vi "GUI Init.vi"(8 "error in (no error)":errorcluster, 10 "GUI Refs":T1, 11 "View Model":T2) -> (0 "error out":errorcluster, 3 "View Model":T2)   [LabVIEW 2017]
doc: "Initialize all GUI Arrays of all used modules"
uses:
  View Model/Controls/View Model.ctl
  View Model/Controls/Shared Model.ctl
  Error Handler/Controls/Error Model.ctl
  Error Handler/Controls/Error Event.ctl
  Error Handler/Controls/Error Type.ctl
  Controller/Controls/Controller Model.ctl
  Controller/Controls/Controller Event.ctl
  Controller/Controls/Controller Command.ctl
  Controller/Controls/Controller Overhead.ctl
  Real-Time/RT Status.ctl
  Real-Time/RT Loop Status.ctl
  Controller/Controls/Controller NStream.ctl
  Controller/Controls/Controller Timer Data.ctl
  Controller/Controls/Controller DAQ Data.ctl
  TDMS Logger/Controls/TDMS Model.ctl
  TDMS Logger/Controls/TDMS Event.ctl
  TDMS Logger/Controls/TDMS Command.ctl
  TDMS Logger/Controls/TDMS Overhead.ctl
  TDMS Logger/Controls/TDMS ChanProperties.ctl
  TDMS Logger/Controls/TDMS DAQ Data.ctl
  Controls/GUI Referencies.ctl
  Controls/TDMS_GUI_Cluster.ctl
  Controls/AIMV_GUI_Cluster.ctl
  Controls/AOM_GUI_Cluster.ctl
  Controls/Discrete_GUI_Cluster.ctl
  GUI Init - DOM6.vi
  GUI Init - DIM4.vi
  GUI Init - DIM3.vi
  GUI Init - AIMC.vi
  GUI Init - AIMV.vi
  GUI Init - AOM.vi
  GUI Init - DOM7.vi
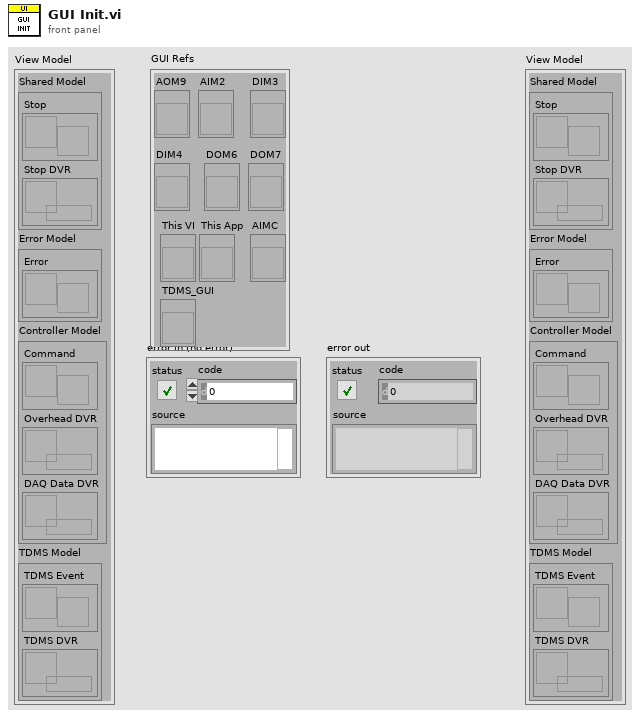
[diagram p1: front panel]
types:
  T1 = typedef "GUI Referencies.ctl" = cluster{"This VI":refnum<vi>, "This App":refnum<vi>, "DIM3":refnum<vi>, "DIM4":refnum<vi>, "DOM6":refnum<vi>, "DOM7":refnum<vi>, "AOM9":refnum<vi>, "AIM2":refnum<vi>, "AIMC":refnum<vi>, "TDMS_GUI":refnum<vi>}
  T2 = typedef "View Model.ctl" = cluster{"Shared Model":T3, "Error Model":T4, "Controller Model":T5, "TDMS Model":T6}
  T3 = typedef "Shared Model.ctl" = cluster{"Stop":refnum<user-event>, "Stop DVR":refnum<data-value>}
  T4 = typedef "Error Model.ctl" = cluster{"Error":refnum<user-event>}
  T5 = typedef "Controller Model.ctl" = cluster{"Command":refnum<user-event>, "Overhead DVR":refnum<data-value>, "DAQ Data DVR":refnum<data-value>}
  T6 = typedef "TDMS Model.ctl" = cluster{"TDMS Event":refnum<user-event>, "TDMS DVR":refnum<data-value>}
  T7 = enum8{"Enabled", "Disabled", "Disabled and Grayed Out"}
  T8 = typedef "Controller DAQ Data.ctl" = cluster{"AOM data":dbl[], "AIMV data":dbl[], "AIMC data":dbl[], "DOM data":dbl[], "DIM data":dbl[], "AOM timestamp":dbl, "AIMV timestamp":dbl, "AIMC timestamp":dbl, "DOM timestamp":dbl, "DIM timestamp":dbl}
  T9 = typedef "AIMV_GUI_Cluster.ctl" = cluster{"Ch.name":string, "Ch.value":dbl, "Ch.range":string, "Num":string}
  T10 = typedef "Discrete_GUI_Cluster.ctl" = cluster{"Ch.name":string, "Ch.state":bool, "Num":string}
  T11 = typedef "AOM_GUI_Cluster.ctl" = cluster{"Ch.name":string, "Ch.value":dbl, "Ch.mode":enum16{"0-5 V", "+/-10 V", "0-5 mA", "4-20 mA"}, "Num":string}
  T12 = typedef "TDMS ChanProperties.ctl" = cluster{"AOM9":string[][], "AIM2":string[][], "DIM3":string[][], "DIM4":string[][], "DOM6":string[][], "DOM7":string[][]}
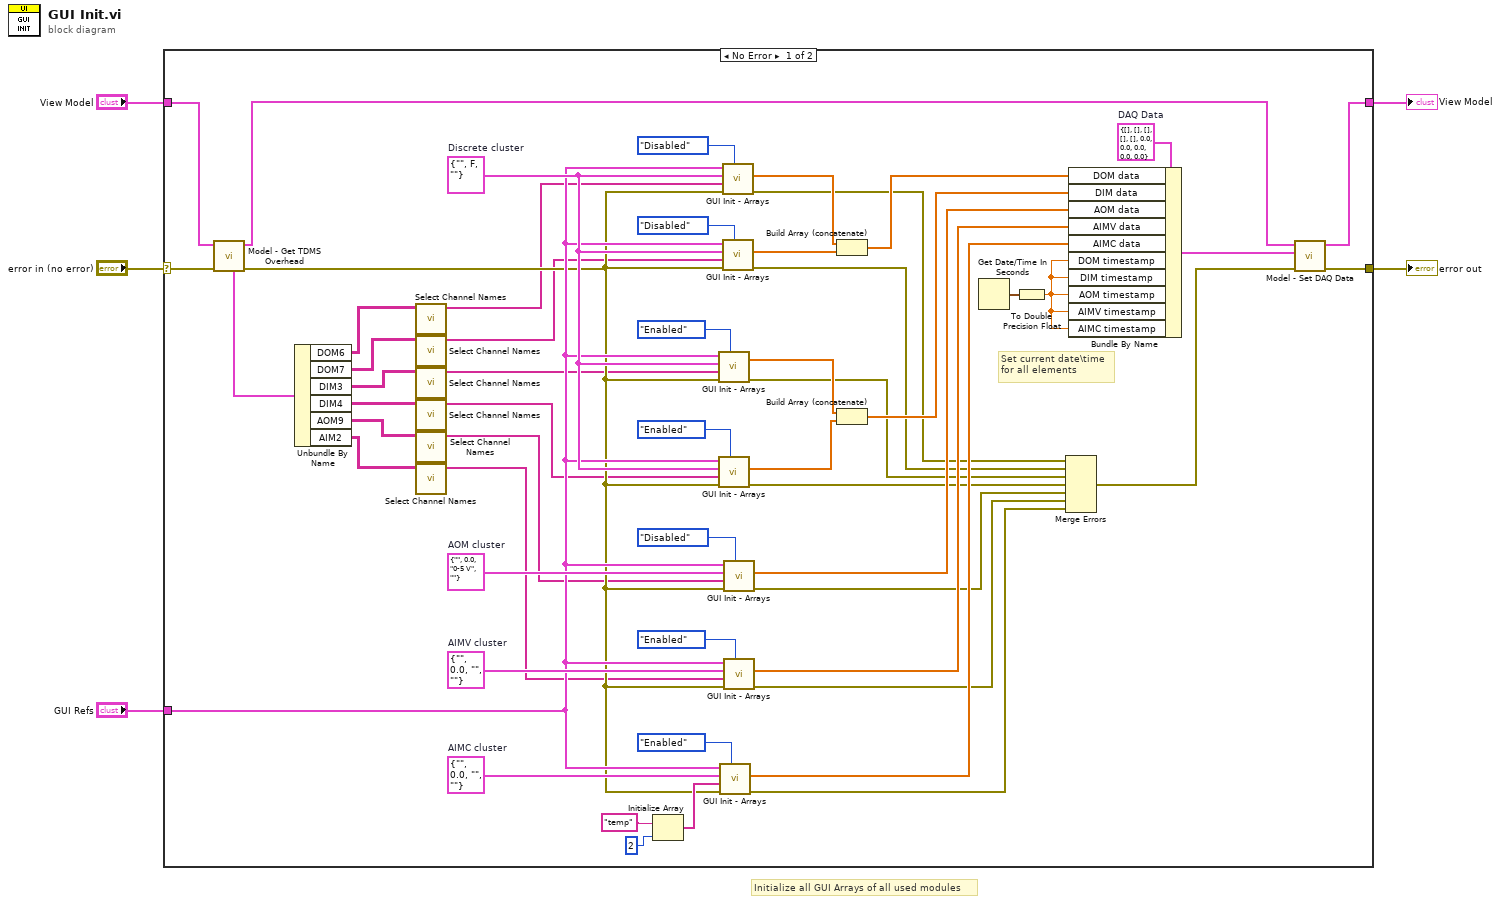
[diagram p0: block diagram]
diagram:
  # "Initialize all GUI Arrays of all used modules"
  n1 = case shown="No Error" "error in (no error)" {
    selector: "error in (no error)" -> [w33 w61]
    tunnel: [w51 w61] -> w4
    tunnel: "View Model" -> [w36 w62]
    tunnel: [w53 w62] -> w2
    tunnel: "GUI Refs" -> [w37 _]
    frame No Error {
      w57 = T8 {"AOM data"=[], "AIMV data"=[], "AIMC data"=[], "DOM data"=[], "DIM data"=[], "AOM timestamp"=0.0, "AIMV timestamp"=0.0, "AIMC timestamp"=0.0, "DOM timestamp"=0.0, "DIM timestamp"=0.0}  # DAQ Data
      w59 = T9 {"Ch.name"="", "Ch.value"=0.0, "Ch.range"="", "Num"=""}  # AIMV cluster
      w47 = T10 {"Ch.name"="", "Ch.state"=FALSE, "Num"=""}  # Discrete cluster
      w60 = T11 {"Ch.name"="", "Ch.value"=0.0, "Ch.mode"=enum."0-5 V", "Num"=""}  # AOM cluster
      w58 = T9 {"Ch.name"="", "Ch.value"=0.0, "Ch.range"="", "Num"=""}  # AIMC cluster
      # "Set current date\\time\nfor all elements"
      n2 = call "Model - Get TDMS Overhead.vi"("error in (no error)"=w33, "View Model"=w36) -> ("error out"=w32:errorcluster, "View Model"=w35:T2, "ChProps"=w34:T12)  [unwired: 4 in, 3 out]
      n3 = Unbundle By Name(w34) -> ("DOM6"=w17:string[][], "DOM7"=w16:string[][], "DIM3"=w15:string[][], "DIM4"=w14:string[][], "AOM9"=w13:string[][], "AIM2"=w12:string[][])
      n4 = call "Select Channel Names.vi"("2D Channel Params"=w17) -> ("Ch.Description -1"=w11:string[])  [unwired: 8 in, 2 out]
      n5 = call "Select Channel Names.vi"("2D Channel Params"=w16) -> ("Ch.Description -1"=w10:string[])  [unwired: 8 in, 2 out]
      n6 = call "Select Channel Names.vi"("2D Channel Params"=w15) -> ("Ch.Description -1"=w9:string[])  [unwired: 8 in, 2 out]
      n7 = call "Select Channel Names.vi"("2D Channel Params"=w14) -> ("Ch.Description -1"=w8:string[])  [unwired: 8 in, 2 out]
      n8 = call "Select Channel Names.vi"("2D Channel Params"=w13) -> ("Ch.Description -1"=w7:string[])  [unwired: 8 in, 2 out]
      n9 = call "Select Channel Names.vi"("2D Channel Params"=w12) -> ("Ch.Description -1"=w6:string[])  [unwired: 8 in, 2 out]
      n10 = Initialize Array("temp" ("Ch.range"), 2 ("dimension size")) -> (w44:string[])
      n11 = call-poly "GUI Init - Arrays.vi"("Disabled"=T7."Enabled", "error in (no error)"=w32, "Ch.names"=w9, "Cluster"=w47, "GUI Refs"=w37) -> ("error out"=w20:errorcluster, "Data"=w39:dbl[])  [unwired: 4 in, 1 out]
      n12 = call-poly "GUI Init - Arrays.vi"("Disabled"=T7."Enabled", "error in (no error)"=w32, "Ch.names"=w8, "Cluster"=w47, "GUI Refs"=w37) -> ("error out"=w21:errorcluster, "Data"=w40:dbl[])  [unwired: 4 in, 1 out]
      n13 = call-poly "GUI Init - Arrays.vi"("Disabled"=T7."Enabled", "error in (no error)"=w32, "Ch.names"=w44, "Cluster"=w58, "GUI Refs"=w37) -> ("error out"=w31:errorcluster, "Data"=w50:dbl[])  [unwired: 4 in, 1 out]
      n14 = call-poly "GUI Init - Arrays.vi"("Disabled"=T7."Disabled", "error in (no error)"=w32, "Ch.names"=w11, "Cluster"=w47, "GUI Refs"=w37) -> ("error out"=w18:errorcluster, "Data"=w43:dbl[])  [unwired: 4 in, 1 out]
      n15 = call-poly "GUI Init - Arrays.vi"("Disabled"=T7."Disabled", "error in (no error)"=w32, "Ch.names"=w10, "Cluster"=w47, "GUI Refs"=w37) -> ("error out"=w19:errorcluster, "Data"=w42:dbl[])  [unwired: 4 in, 1 out]
      n16 = call-poly "GUI Init - Arrays.vi"("Disabled"=T7."Disabled", "error in (no error)"=w32, "Ch.names"=w7, "Cluster"=w60, "GUI Refs"=w37) -> ("error out"=w29:errorcluster, "Data"=w48:dbl[])  [unwired: 4 in, 1 out]
      n17 = call-poly "GUI Init - Arrays.vi"("Disabled"=T7."Enabled", "error in (no error)"=w32, "Ch.names"=w6, "Cluster"=w59, "GUI Refs"=w37) -> ("error out"=w30:errorcluster, "Data"=w49:dbl[])  [unwired: 4 in, 1 out]
      n18 = Build Array (concatenate)(w43, w42) -> (w41:dbl[])
      n19 = Build Array (concatenate)(w39, w40) -> (w38:dbl[])
      n20 = Get Date/Time In Seconds() -> (seconds since 1Jan1904=w56:timestamp)
      n21 = To Double Precision Float(number=w56) -> (double precision float=w55:dbl)
      n22 = Merge Errors(w18, w19, w20, w21, w29, w30, w31) -> (w52:errorcluster)
      n23 = Bundle By Name(cluster=w57, "DOM data"=w41, "DIM data"=w38, "AOM data"=w48, "AIMV data"=w49, "AIMC data"=w50, "DOM timestamp"=w55, "DIM timestamp"=w55, "AOM timestamp"=w55, "AIMV timestamp"=w55, "AIMC timestamp"=w55) -> (w54:T8)
      n24 = call "Model - Set DAQ Data.vi"("error in (no error)"=w52, "DAQ Data"=w54, "View Model"=w35) -> ("error out"=w51:errorcluster, "View Model"=w53:T2)  [unwired: 7 in]
    }
    frame Error {
    }
  }
  "View Model" <- w2
  "error out" <- w4
